vi "Profile 2 Possible IDs.vi"(7 "Profile Step":string[](array[string]), 11 "StepIndex":i32) -> (8 "Step ID":string)   [LabVIEW 2013]
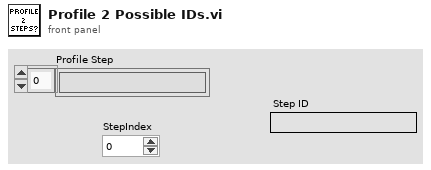
[diagram p1: front panel]
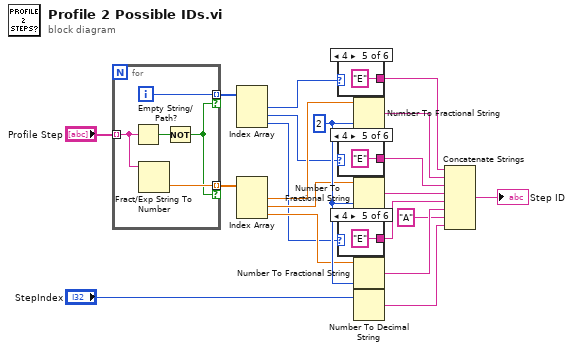
[diagram p0: block diagram]
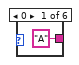
[diagram p2: hidden frame]
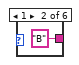
[diagram p3: hidden frame]
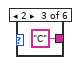
[diagram p4: hidden frame]
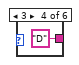
[diagram p5: hidden frame]
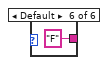
[diagram p6: hidden frame]
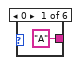
[diagram p7: hidden frame]
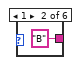
[diagram p8: hidden frame]
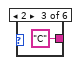
[diagram p9: hidden frame]
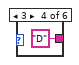
[diagram p10: hidden frame]
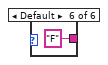
[diagram p11: hidden frame]
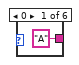
[diagram p12: hidden frame]
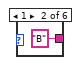
[diagram p13: hidden frame]
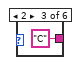
[diagram p14: hidden frame]
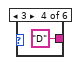
[diagram p15: hidden frame]
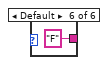
[diagram p16: hidden frame]
diagram:
  w16 = i16 2 ("width (-)")
  n1 = for {
    tunnel: "Profile Step" -> [w23] mode=indexing
    tunnel: [w24] -> w19 mode=indexing if=w21
    tunnel: [w22] -> w18 mode=indexing if=w21
    i -> [w24]
    n2 = Empty String/Path?(string/path=w23) -> (empty?=w25:bool)
    n3 = Fract/Exp String To Number(string=w23) -> (number=w22:dbl)  [unwired: 3 in, 1 out]
    n4 = Not(x=w25) -> (.not. x?=w21:bool)
  }
  n5 = Index Array(array=w19) -> (element #1=w9:i32, element #2=w7:i32, element #3=w2:i32)  [unwired: 3 in]
  n6 = Index Array(array=w18) -> (element #1=w8:dbl, element #2=w6:dbl, element #3=w5:dbl)  [unwired: 3 in]
  n7 = case shown="4" w9 {
    tunnel: ["A" "B" "C" "D" "E" "F"] -> w15
    frame 0 {
    }
    frame 1 {
    }
    frame 2 {
    }
    frame 3 {
    }
    frame 4 {
    }
    frame Default {
    }
  }
  n8 = case shown="4" w7 {
    tunnel: ["A" "B" "C" "D" "E" "F"] -> w13
    frame 0 {
    }
    frame 1 {
    }
    frame 2 {
    }
    frame 3 {
    }
    frame 4 {
    }
    frame Default {
    }
  }
  n9 = case shown="4" w2 {
    tunnel: ["A" "B" "C" "D" "E" "F"] -> w1
    frame 0 {
    }
    frame 1 {
    }
    frame 2 {
    }
    frame 3 {
    }
    frame 4 {
    }
    frame Default {
    }
  }
  n10 = Number To Fractional String(number=w8, precision (6)=w16) -> (F-format string=w14:string)  [unwired: 2 in]
  n11 = Number To Fractional String(number=w6, precision (6)=w16) -> (F-format string=w12:string)  [unwired: 2 in]
  n12 = Number To Fractional String(number=w5, precision (6)=w16) -> (F-format string=w17:string)  [unwired: 2 in]
  n13 = Number To Decimal String(number="StepIndex") -> (decimal integer string=w10:string)  [unwired: 1 in]
  n14 = Concatenate Strings(w15, w14, w13, w12, w1, w17, "A" ("string"), w10) -> (→"Step ID":string)
